vi "Thermocouple Read v1_1.vi"() -> (0 "Cluster":T1 {"Resevoir Temp" format="%.6g"; "Inlet Dry Bulb Temp" format="%.6g"; "Inlet Wet Bulb Temp" format="%.6g"; "Outlet Wet Bulb Temp" format="%.6g"; "Outlet Dry Bulb Temp" format="%.6g"; "Inlet Water Temp" format="%.6g"; "Outlet Water Temp" format="%.6g"})   [LabVIEW 2012]
panel:
  in  "Enum":enum16{"1", "10", "100", "1000"}(ring)
  in  "stop":bool
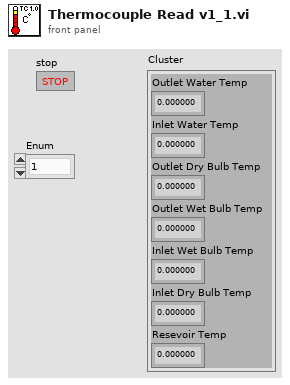
[diagram p1: front panel]
types:
  T1 = cluster{"Outlet Water Temp":dbl, "Inlet Water Temp":dbl, "Outlet Dry Bulb Temp":dbl, "Outlet Wet Bulb Temp":dbl, "Inlet Wet Bulb Temp":dbl, "Inlet Dry Bulb Temp ":dbl, "Resevoir Temp":dbl}
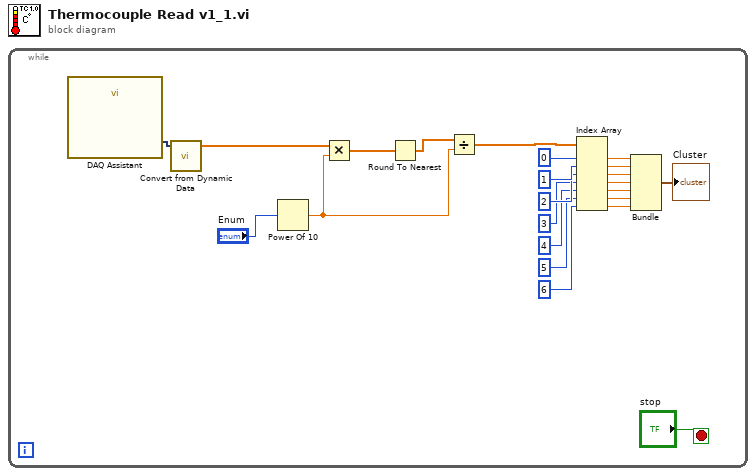
[diagram p0: block diagram]
diagram:
  n1 = while {
    stop <- "stop" stop-if-true
    n2 = call "DAQ Assistant"() -> ("data"=w23:dynamicdata)  [unwired: 17 in, 2 out]
    n3 = call "Convert from Dynamic Data"("Dynamic Data Type"=w23) -> ("Array"=w22:dbl[])  [unwired: 3 in]
    n4 = Power Of 10(x="Enum") -> (10^x=w8:dbl)
    n5 = Multiply(x=w22, y=w8) -> (x*y=w13:dbl[])
    n6 = Round To Nearest(number=w13) -> (nearest integer value=w12:dbl[])
    n7 = Divide(x=w12, y=w8) -> (x/y=w11:dbl[])
    n8 = Index Array(array=w11, index #1=0, index #2=1, index #3=2, index #4=3, index #5=4, index #6=5, index #7=6) -> (element #1=w7:dbl, element #2=w6:dbl, element #3=w5:dbl, element #4=w4:dbl, element #5=w3:dbl, element #6=w2:dbl, element #7=w1:dbl)
    n9 = Bundle(w7, w6, w5, w4, w3, w2, w1) -> (→"Cluster":cluster{dbl, dbl, dbl, dbl, dbl, dbl, dbl})  [unwired: 1 in]
  }
